vi "Get Autonomous Data.vi"(11 "Autonomous Selectin":string="Robot Right Switch Left") -> (3 "Autonomous Data Selected":T1(array[cluster]))   [LabVIEW 2017]
uses:
  Framework/Robot Global Data.vi
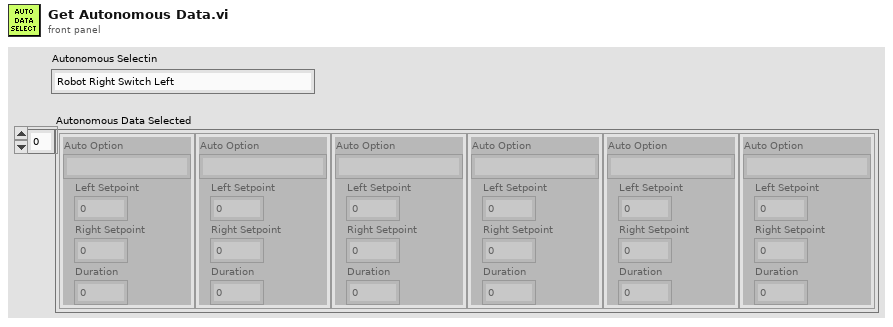
[diagram p1: front panel]
types:
  T1 = cluster{"Auto Option":string, "Left Setpoint":dbl, "Right Setpoint":dbl, "Duration":dbl}[]
  T2 = cluster{"Auto Option":string, "Left Setpoint":dbl, "Right Setpoint":dbl, "Duration":dbl}[][]
  T3 = cluster{"Auto Option":string, "Left Setpoint":dbl, "Right Setpoint":dbl, "Duration":dbl}
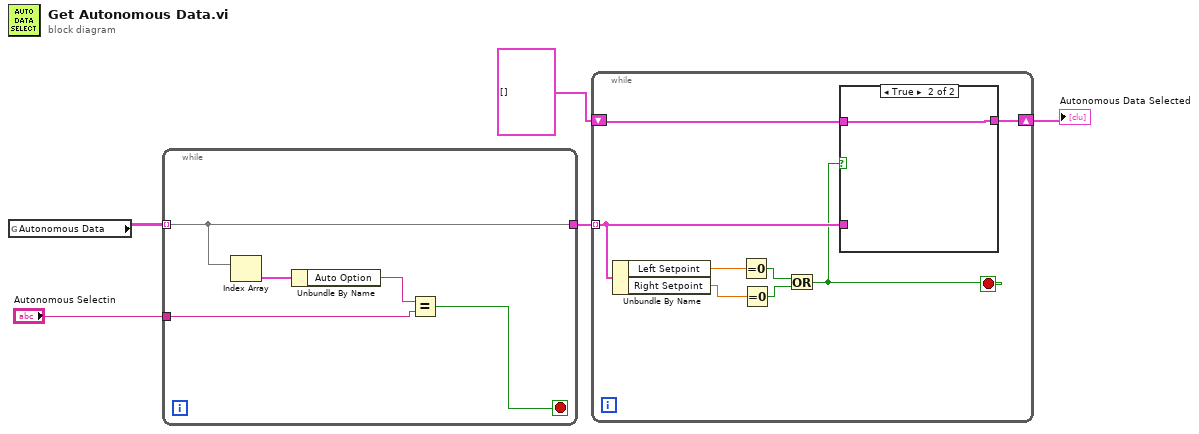
[diagram p0: block diagram]
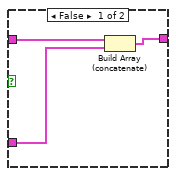
[diagram p2: hidden frame]
diagram:
  n1 = global read "Robot Global Data.vi" "Autonomous Data"() -> (w5:T2)
  n2 = while {
    tunnel: w5 -> [w6] mode=indexing
    tunnel: "Autonomous Selectin" -> [w8]
    tunnel: [w6] -> w4
    stop <- w7 stop-if-true
    n3 = Index Array(array=w6) -> (element=w10:T3)  [unwired: 1 in]
    n4 = Unbundle By Name(w10) -> ("Auto Option"=w9:string)
    n5 = Equal?(x=w9, y=w8) -> (x = y?=w7:bool)
  }
  n6 = while {
    tunnel: w4 -> [w13] mode=indexing
    shift-right: [w12] -> w2
    shift-left: T1 [] -> [w14]
    stop <- w11 stop-if-true
    n7 = Unbundle By Name(w13) -> ("Left Setpoint"=w18:dbl, "Right Setpoint"=w15:dbl)
    n8 = Equal To 0?(x=w18) -> (x = 0?=w16:bool)
    n9 = Equal To 0?(x=w15) -> (x = 0?=w17:bool)
    n10 = Or(x=w16, y=w17) -> (x .or. y?=w11:bool)
    n11 = case shown="True" w11 {
      tunnel: w14 -> [w21 w22]
      tunnel: w13 -> [w20 _]
      tunnel: [w19 w22] -> w12
      frame False {
        n12 = Build Array (concatenate)(w21, w20) -> (w19:T1)
      }
      frame True {
      }
    }
  }
  "Autonomous Data Selected" <- w2
